vi "ta_calc_diff.vi"(11 "data in":dbl[][](array[numeric])) -> (1 "diff":dbl[](array[numeric]), 2 "unpumped":dbl[](array[numeric]), 3 "pumped":dbl[](array[numeric]))   [LabVIEW 2019]
uses:
  <vilib>/Analysis/baseanly.llb/Mean (DBL).vi
  <vilib>/Analysis/NI_AALBase.lvlib
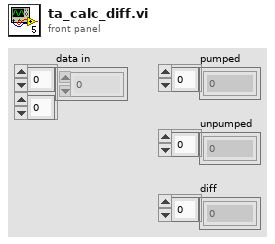
[diagram p1: front panel]
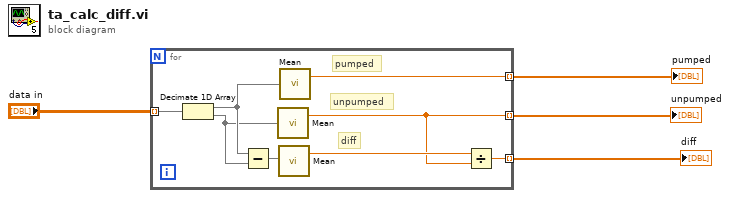
[diagram p0: block diagram]
diagram:
  n1 = for {
    tunnel: "data in" -> [w5] mode=indexing
    tunnel: [w6] -> w3 mode=indexing
    tunnel: [w7] -> w2 mode=indexing
    tunnel: [w9] -> w1 mode=indexing
    # "diff"
    # "unpumped"
    # "pumped"
    n2 = Decimate 1D Array(w5) -> (w11:dbl[], w10:dbl[])
    n3 = Subtract(x=w11, y=w10) -> (x-y=w12:dbl[])
    n4 = call-poly <vilib>:"Mean.vi"("X"=w10) -> ("mean"=w7:dbl)  [unwired: 1 out]
    n5 = call-poly <vilib>:"Mean.vi"("X"=w12) -> ("mean"=w8:dbl)  [unwired: 1 out]
    n6 = call-poly <vilib>:"Mean.vi"("X"=w11) -> ("mean"=w9:dbl)  [unwired: 1 out]
    n7 = Divide(x=w8, y=w7) -> (x/y=w6:dbl)
  }
  "diff" <- w3
  "unpumped" <- w2
  "pumped" <- w1
